vi "Pre Launch Init.vi"(11 "Trace Controller in":refnum<class "Trace Controller.lvclass">) -> (0 "error out":errorcluster, 3 "Trace Controller out":refnum<class "Trace Controller.lvclass">)   [LabVIEW 2014, in "Robot Actor Framework.lvlib" / "Trace.lvlib" / "Trace Controller.lvclass"]
doc: "(<B>Filename</B>: Actor Framework.lvlib:Actor.lvclass:Pre Launch Init.vi)\n\nDefines behavior that occurs after the Launch Actor method is invoked but before the actor's Actor Core method begins running.\n\nThe Pre Launch Init method is guaranteed to finish before the Launch Actor method returns to its caller and before the actor itself receives any messages. Any references that the Pre Launch Init method obtains are guaranteed to have the same lifetime as the actor itself. Any errors that the Pre Launch Init method returns will abort the launch.\n\nBy default, this method does nothing. A descendant class may override it to define behavior."
uses:
  Trace Controller.lvclass
  Trace Class/Trace.lvclass
  Trace Controller.lvclass/Trace Controller.ctl
  System Actor/System Actor Class/System Actor.lvclass
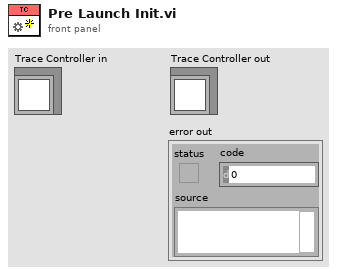
[diagram p1: front panel]
types:
  T1 = enum16{"open", "replace", "create", "open or create", "replace or create", "replace or create with confirmation"}
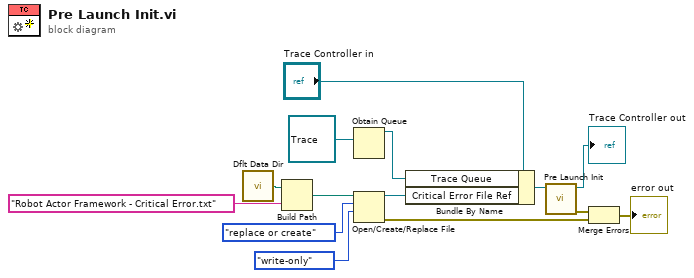
[diagram p0: block diagram]
diagram:
  n1 = call <vilib>:"Dflt Data Dir.vi"() -> ("App:Default Data Directory"=w1:path)
  n2 = Build Path(base path=w1, name or relative path="Robot Actor Framework - Critical Error.txt") -> (appended path=w4:path)
  n3 = Obtain Queue(element data type=refnum<class "Trace.lvclass"> refnum ("Robot Actor Framework.lvlib:Trace.lvlib:Trace.lvclass")) -> (queue out=w10:refnum<queue>)  [unwired: 4 in, 2 out]
  n4 = Open/Create/Replace File(file path (use dialog)=w4, operation (0:open)=T1."replace or create", access (0:read/write)=enum16{"read/write", "read-only", "write-only"}."write-only") -> (refnum out=w8:refnum<file>, error out=w2:errorcluster)  [unwired: 3 in, 1 out]
  n5 = Bundle By Name(cluster="Trace Controller in", "Trace Queue"=w10, "Critical Error File Ref"=w8) -> (w11:refnum<class "Trace Controller.lvclass">)
  n6 = call-parent "Pre Launch Init.vi"("System Actor in"=w11) -> ("error out"=w14:errorcluster, "System Actor out"=→"Trace Controller out":refnum<class "Trace Controller.lvclass">)  [unwired: 9 in]
  n7 = Merge Errors(w14, w2) -> (→"error out":errorcluster)
